vi "GetMyAttribute.vi"(8 "error in (no error)":errorcluster, 11 "reference in":refnum<class "MyPropertyClass_LV2009.lvclass">) -> (0 "error out":errorcluster, 2 "MyAttribute":dbl, 3 "reference out":refnum<class "MyPropertyClass_LV2009.lvclass">)   [LabVIEW 2017, in "MyPropertyClass_LV2009.lvclass"]
doc: "Access to MyAttribute"
uses:
  MyPropertyClass_LV2009.lvclass
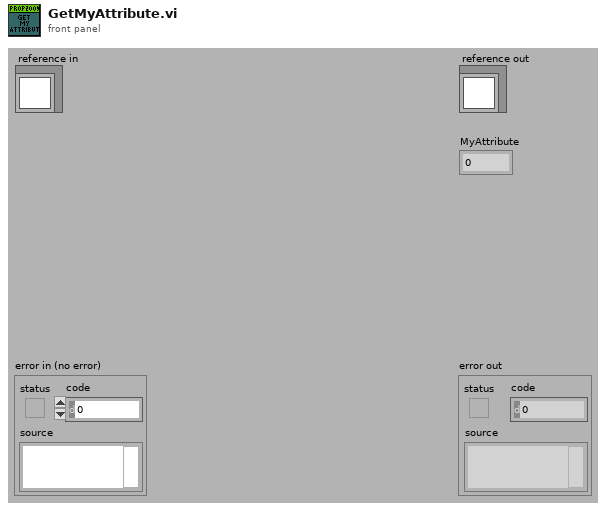
[diagram p1: front panel]
types:
  T1 = typedef "MyPropertyClass_LV2009.lvclass/ObjectAttributesRef.ctl" = refnum<data-value>
  T2 = typedef "MyPropertyClass_LV2009.lvclass/ObjectAttributes.ctl" = cluster{"MyAttribute":dbl, "Name":string}
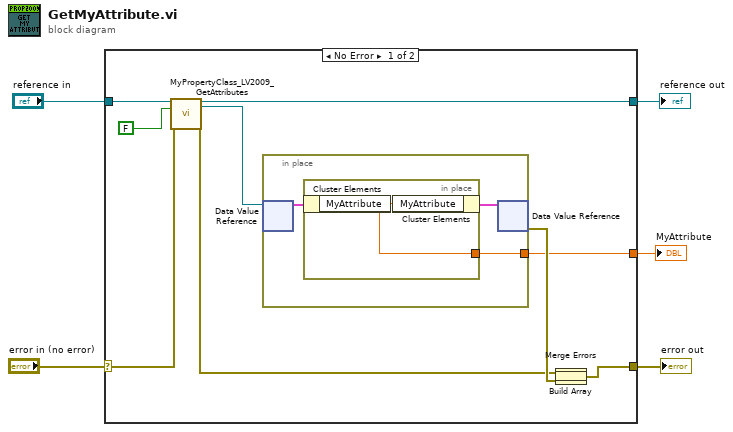
[diagram p0: block diagram]
diagram:
  n1 = case shown="No Error" "error in (no error)" {
    selector: "error in (no error)" -> [w15 w21]
    tunnel: [w9 w21] -> w4
    tunnel: [w14 w20] -> w2
    tunnel: "reference in" -> [w13 w20]
    tunnel: [w7 _] -> w1
    frame No Error {
      n2 = call "MyPropertyClass_LV2009_GetAttributes.vi"("reference in"=w13, "return data? (T)"=FALSE, "error in (no error)"=w15) -> ("reference out"=w14:refnum<class "MyPropertyClass_LV2009.lvclass">, "attributes ref"=w8:T1, "error out"=w10:errorcluster)  [unwired: 13 in, 1 out]
      n3 = in-place {
        in-place-border: [w16] -> w7
        n4 = in-place-dvr #1(w8) -> (w17:T2)  [unwired: 1 out]
        n5 = in-place {
          in-place-border: [w19] -> w16
          n6 = in-place-cluster #2(w17) -> ("MyAttribute"=w19:dbl)
          n7 = in-place-cluster #2("MyAttribute"=w19) -> (w18:T2)
        }
        n8 = in-place-dvr #1(w18) -> (w11:errorcluster)  [unwired: 1 out]
      }
      n9 = Build Array(w10, w11) -> (w6:errorcluster[])
      n10 = Merge Errors(w6) -> (w9:errorcluster)
    }
    frame Error {
    }
  }
  "error out" <- w4
  "reference out" <- w2
  "MyAttribute" <- w1
